vi "Main v1.9.vi"() -> ()   [LabVIEW 2017]
doc: "v0.85:\n- Counts for rejects and total\n\nv0.5:\n\n- Added Reject to Manual Mode\n- Send reject pallet cluster during manual mode\n- Run continuous manual happens only when no error has occured"
uses:
  Controls/Main Tabs v0.1.ctl
  Controls/Auto.ctl
  RT/Controls/Auto Delays.ctl
  RT/Controls/Auto Times.ctl
  support/Controls/General Para.ctl
  Controls/UI Data.ctl
  Controls/AVL Auto Time.ctl
  support/Controls/Auto Stats.ctl
  Controls/Logging FGV.ctl
  support/Message Queue/Enqueue Message (Single).vi
  GV/Maintenance GV.vi
  <vilib>/Utility/error.llb/Error Cluster From Error Code.vi
  <vilib>/ErrorRing/Error Ring.xnode
  support/Message Queue/Message Queue.lvlib
  support/User Event - Stop/User Event - Stop.lvlib
panel:
  out "Rejects 2":u32 caption="Rejects"
  in  "Reset MCount":bool
  out "Output Count":u32 caption="Output\nCount"
  out "OEE":dbl format="%#.1f"
  out "QUA":dbl=100.0 min=0.0 max=100.0 step=0.1
  in  "Ideal Time":dbl=2.0 min=0.0 max=100.0 step=0.1
  in  "AVL":dbl=100.0 min=0.0 max=100.0 step=0.1
  out "PRF":dbl=100.0 min=0.0 max=100.0 step=0.1
  out "path":path
  in  "General Para 2":T1={"Max. Cons."=5.0, "Offset 1"=0.0, "Offset 2"=0.0, "Offset 3"=0.0, "Offset 4"=-0.6, "OutputPause"=500.0, "RejectPause"=500.0} caption="General Para" {"Offset 4" format="%.2f"; "Offset 3" format="%.2f"; "Offset 2" format="%.2f"; "Offset 1" format="%.2f"}
  in  "Auto Para 2":T2={"Agitator Delays"=[250, 600], "TF Delays"=[400, 800, 2, 8000], "Insertion Delays"=[100, 400], "Cutting Delays"=[200, 300, 50], "PF Delays"=[300, 8000], "Measur. Delays"=[200.0, 188.9, 1.0], "Reject Delays"=[500], "BF Delays"=[1000, 1000]}
  out "Shutdown?":bool
  in  "Reject Pallets":T3
  out "Date-Time":string caption="Dip-Tube Assembly Automation (HMI) v1.6"
  out "Main Tab":T4
  in  "All IOs":bool
  in  "Autocycle":T5
  in  "Manual":bool
  in  "Parameters":bool
  in  "Maintenance":bool
  in  "General Para":T1={"Max. Cons."=5.0, "Offset 1"=0.0, "Offset 2"=0.0, "Offset 3"=0.0, "Offset 4"=0.0, "OutputPause"=0.0, "RejectPause"=0.0} {"Offset 4" format="%.2f"; "Offset 3" format="%.2f"; "Offset 2" format="%.2f"; "Offset 1" format="%.2f"}
  in  "BF Para":cluster{"Delay 1":u32, "Delay 2":u32}={"Delay 1"=1000, "Delay 2"=1000}
  in  "Reject Para":cluster{"Delay":u32}={"Delay"=400}
  in  "PF Para":cluster{"Delay 1":u32, "Delay 2":u32}={"Delay 1"=1000, "Delay 2"=1000}
  in  "Tube Feeder Para":T6={"Delay"=400, "Delay 2"=250, "Max Attempts"=250, "Timeout"=8000} caption="TF Para"
  in  "Agitator Para":cluster{"Delay 1":u32, "Delay 2":u32}={"Delay 1"=400, "Delay 2"=250}
  in  "Insertion Para":cluster{"Delay 1":u32, "Delay 2":u32}={"Delay 1"=1000, "Delay 2"=1000}
  in  "Save Para":bool
  in  "Home Para":bool
  in  "Cutting Para":T7={"Delay"=400, "Delay 2"=250, "Delay 3"=250}
  in  "Meas. Para":T8={"Delay"=500.0, "Mean Length"=188.9, "Tolerance"=1.0}
  in  "Enable BF?":bool
  in  "Enable Agitate?":bool
  in  "Enable Reject?":bool
  in  "Toggle Motor":bool
  in  "Continuous?":bool
  in  "Enable Measure?":bool
  in  "Enable Index?":bool
  in  "Enable PF?":bool
  in  "Manual Para":T2={"Agitator Delays"=[400, 250], "TF Delays"=[700, 800, 2], "Insertion Delays"=[100, 500], "Cutting Delays"=[300, 300, 100], "PF Delays"=[250, 30000], "Measur. Delays"=[500.0, 188.9, 1.0], "Reject Delays"=[500], "BF Delays"=[1000, 1000]}
  in  "Enable Cutting?":bool
  in  "Enable Insertion?":bool
  in  "Run Manual":bool
  in  "Enable TF?":bool
  in  "Home Manual":bool
  out "Status 2":T10
  out "Measurements":T11 {"Height 1" format="%#.2f"; "Height 2" format="%#.2f"; "Height 3" format="%#.2f"; "Height 4" format="%#.2f"}
  in  "ResetRejectCount":bool
  in  "ResetGoodCount":bool
  out "RejectPause":u32 caption="Reject Parts"
  out "GoodPause":u32 caption="Good Parts"
  in  "End Cycle":bool
  out "Statuses":string[][](table)
  in  "All IO":bool
  in  "Stats":bool
  in  "Home AC":bool
  out "Status":string
  out "Good":u32 format="%06.0f"
  out "Cycle Time":dbl format="%0.2f"
  out "Rejects":u32 format="%05.0f"
  in  "View Log":bool
  out "Total Count 2":u32 caption="Total Count"
  out "Avg. Time":dbl caption="Avg. Cycle Time (s)" format="%#.3f"
  out "Output Chart":cluster{"Good Parts":u32, "Reject Parts":u32}(graph)
  out "Reject Count":u32
  out "Good Count":u32
  out "Total Time":dbl caption="Effective Cycle Time (s)" format="%#.3f"
  out "Time Chart":T12(graph)
  out "OEE Chart":T13(graph)
  out "Timestamp":string caption="Date & Timestamp"
  out "Latest Measure.":T14 caption="Latest Measurements" {"Length 1 (mm)" format="%#.2f"}
  out "Auto Times":T9
  in  "Back Stats":bool
  out "OEE 2":T13 caption="Latest Measurements" {"AVL" format="%#.1f"; "PRF" format="%#.1f"; "QUA" format="%#.1f"; "OEE" format="%#.1f"}
  out "Measurement Chart":T15(graph)
  in  "Home IOs":bool
  in  "Back IO":bool
  out "IAS 4":dbl format="%#.3f"
  out "IAS 3":dbl format="%#.3f"
  out "IAS 2":dbl format="%#.3f"
  out "IAS 1":dbl format="%#.3f"
  out "DI 1":T16
  out "DI 2":T17
  out "DO 1":T18
  in  "Exit":bool
  in  "Shutdown":bool
  # "HARMONY VISION DIP-TUBE ASSEMBLY AUTOMATION"
  # "Info"
  # "Delays: Time to wait (in milliseconds) after each action pertaining to each spcific station. Generally this timer starts after the required sensor that is expected either goes OFF or goes ON depending on the action. Some stations have multiple delays which are denoted by numbers relative to the sequence of action before the delay.\n\nTimeout: Maximum time allowed (in milliseconds) for a station to complete its actions.\n\nMax Attempts: Maximum number of attempts at retrying gate open/close.\n\nMean Length: Mean length of parts in the current model (in mm)\n\nTolerance: Acceptable deviation from mean length (in mm)\n\nMax Cons.: Maximum number of consecutive tubes missing on a particular pallet (as detected on measurement station) that will trigger an error and cycle stop.\n\nOffset: Offset factor (in mm) added to the measurement result of each probe.\n\nOutputPause & RejectPause: Countdown of number of parts before triggering an Auto-Pause."
  # "Auto-Pause after"
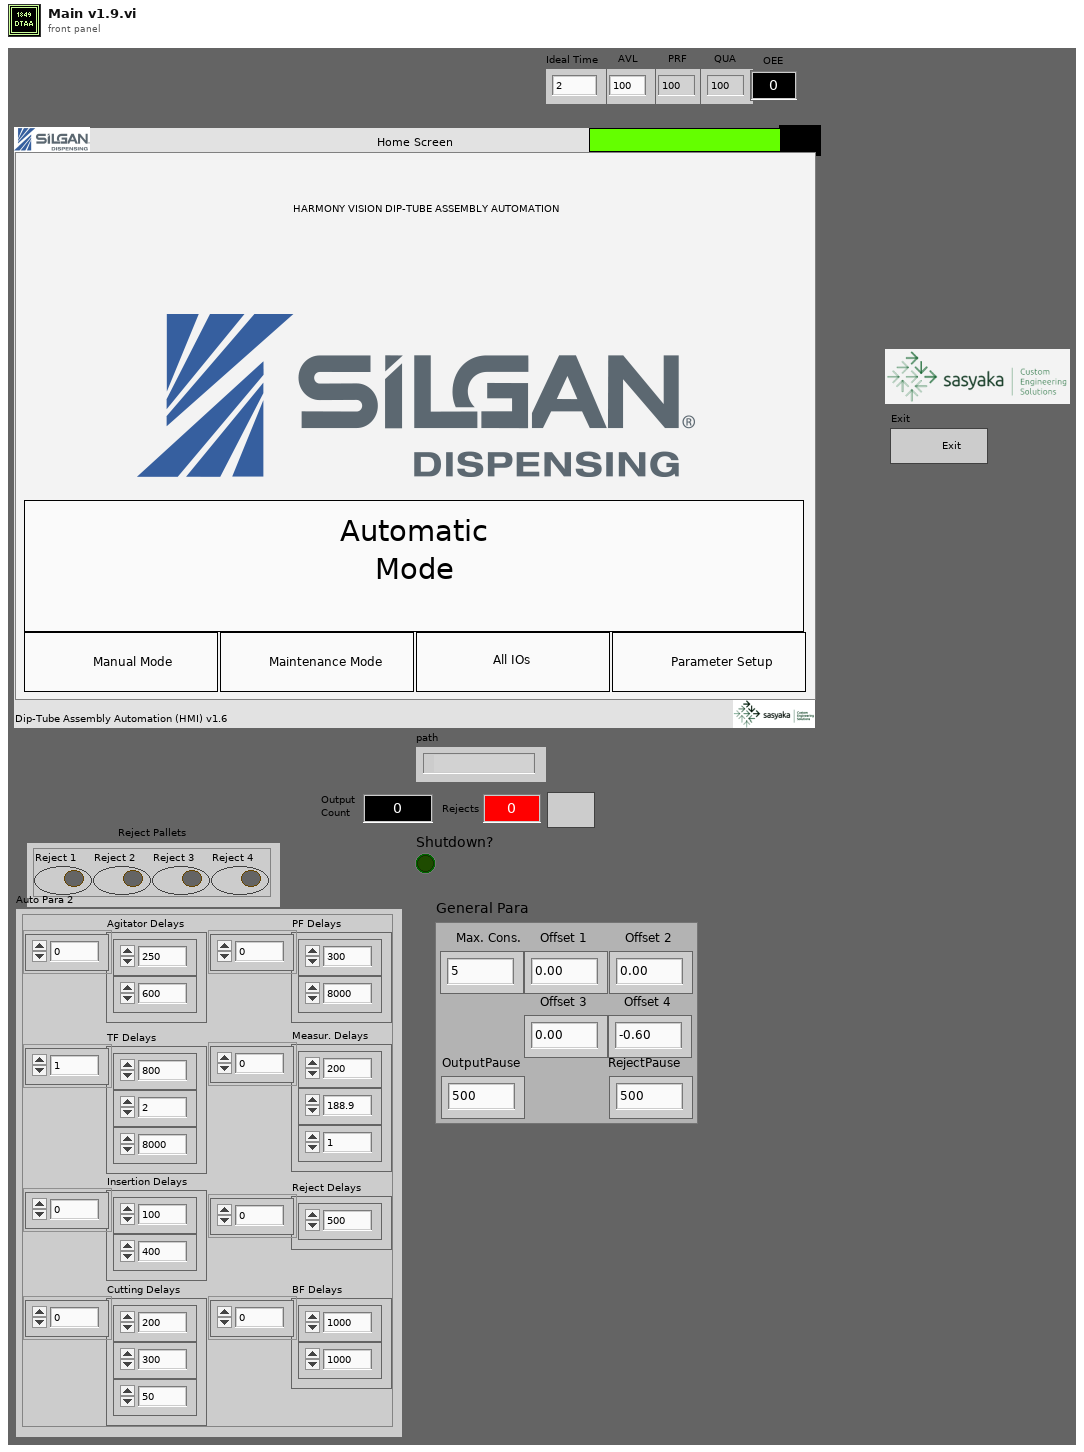
[diagram p1: front panel]
types:
  T1 = typedef "General Para.ctl" = cluster{"Max. Cons.":dbl, "Offset 1":dbl, "Offset 2":dbl, "Offset 3":dbl, "Offset 4":dbl, "OutputPause":dbl, "RejectPause":dbl}
  T2 = typedef "Auto Delays.ctl" = cluster{"Agitator Delays":u32[], "TF Delays":u32[], "Insertion Delays":u32[], "Cutting Delays":u32[], "PF Delays":u32[], "Measur. Delays":dbl[], "Reject Delays":u32[], "BF Delays":u32[]}
  T3 = cluster{"Reject 1":bool, "Reject 2":bool, "Reject 3":bool, "Reject 4":bool}
  T4 = typedef "Main Tabs v0.1.ctl" = enum32{"Home Screen", "Parameter Setup", "Manual Mode", "Autocycle", "Autocycle Statistics", "Autocycle IOs"}
  T5 = typedef "Auto.ctl" = bool
  T6 = cluster{"Delay":u32, "Delay 2":u32, "Max Attempts":u32, "Timeout":u32}
  T7 = cluster{"Delay":u32, "Delay 2":u32, "Delay 3":u32}
  T8 = cluster{"Delay":dbl, "Mean Length":dbl, "Tolerance":dbl}
  T9 = typedef "Auto Times.ctl" = cluster{"Index Time":u32, "TF Time":u32, "Insertion Time":u32, "Cutting Time":u32, "PF Time":u32, "Meas. Time":u32, "Reject Time":u32}
  T10 = cluster{"Auto Times":T9, "error out":errorcluster}
  T11 = cluster{"Height 1":dbl, "Height 2":dbl, "Height 3":dbl, "Height 4":dbl}
  T12 = cluster{"Index":dbl, "TF":dbl, "Insert":dbl, "Cutting":dbl, "PF":dbl, "Measure.":dbl, "Reject":dbl, "Avg. Cycle Time":dbl}
  T13 = cluster{"AVL":dbl, "PRF":dbl, "QUA":dbl, "OEE":dbl}
  T14 = cluster{"Length 1 (mm)":dbl, "Pallet 2 (mm)":dbl, "Pallet 3 (mm)":dbl, "Pallet 4 (mm)":dbl}
  T15 = cluster{"1":dbl, "2":dbl, "3":dbl, "4":dbl, "4":dbl, "4":dbl}
  T16 = cluster{"Machine_ON":bool, "E_stop ":bool, "SW_Pressure":bool, "SW_Start ":bool, "SW_Reset":bool, "SW_Stop":bool, "SW_Door":bool, "RS_Index_Rotary_CW":bool, "RS_Index_Rotary_CCW":bool, "RS_Index_Stopper _Rear":bool, "RS_Index_Output_Separator_Rear":bool, "PES_Index_Pallet_Sensor":bool, "PES_Index_Output_Part Sensor":bool, "ICS_BF_Low_Level_1":bool, "ICS_BF_Low_Level_2":bool, "ICS_BF_Pump_CNVR_Full_1":bool, "ICS_BF_Pump_CNVR_Full_2":bool, "ICS_BF_Pump_CNVR_Full_3":bool, "ICS_BF_Pump_CNVR_Full_4":bool, "PES_PC_Pump Presence_1":bool, "PES_PC_Pump Presence_2":bool, "PES_PC_Pump Presence_3":bool, "PES_PC_Pump Presence_4":bool, "RS_PC_Gating_Front":bool, "PES_Pump_Interference":bool, "PES_TF_Low_Level":bool, "PES_Tube Presence_1":bool, "PES_Tube Presence_2":bool, "PES_Tube Presence_3":bool, "PES_Tube Presence_4":bool, "DI1.30":bool, "DI1.31":bool}
  T17 = cluster{"RS_Agitatator_1_Rear ":bool, "RS_Agitatator_2_Rear ":bool, "RS_TF_Gating CYL_Rear":bool, "RS_Insertion_1_Rear":bool, "RS_Insertion_1_Front":bool, "RS_Insertion _2_Rear":bool, "RS_Insertion _2_Front":bool, "RS_Insertion _3_Rear":bool, "RS_Insertion _3_Front":bool, "RS_Insertion _4_Rear":bool, "RS_Insertion _4_Front":bool, "RS_Insertion_Clamp_Rear":bool, "RS_Cutting_Rear":bool, "RS_Cutting_Clamp _Rear":bool, "RS_Measurement_1_Rear":bool, "RS_Measurement_2_Rear":bool, "RS_Measurement_3_Rear":bool, "RS_Measurement_4_Rear":bool, "DI2.18":bool, "RS_Rejection_1_Rear":bool, "RS_Rejection_2_Rear":bool, "RS_Rejection_3_Rear":bool, "RS_Rejection_4_Rear":bool, "DI2.23":bool, "DI2.24":bool, "DI2.25":bool, "DI2.26":bool, "DI2.27":bool, "DI2.28":bool, "DI2.29":bool, "DI2.30":bool, "DI2.31":bool}
  T18 = cluster{"TL_Red":bool, "TL_Orange":bool, "TL_Green":bool, "TL_Buzzer":bool, "SOL_Index_Rotary_CW":bool, "SOL_Index_Rotary_CCW":bool, "SOL_Index_Stopper_Rear":bool, "SOL_OutputSeparator_Rear":bool, "Bowl  Feeder_ ON 1":bool, "Pump_CNVR_Motor _ON":bool, "SOL_PC_Gating_CYL_Rear":bool, "SOL_Tube_Feed_Agitatator":bool, "SOL_Tube_Feed_Gating_CYL":bool, "SOL_Insertion _CYL":bool, "SOL_Insertion_Clamp_CYL":bool, "SOL_Cutting_CYL":bool, "SOL_Cutting_Clamp_CYL":bool, "SOL_Insertion_Air_Nozzle":bool, "SOL_Measurement_CYL":bool, "DO1.19":bool, "SOL_Rejection CYL_1":bool, "SOL_Rejection CYL_2":bool, "SOL_Rejection CYL_3":bool, "SOL_Rejection CYL_4":bool, "Bowl  Feeder_ ON 2":bool, "SOL_BF_BlowerON":bool, "SOL_BF1_Track1":bool, "SOL_BF1_Track2":bool, "SOL_BF2_Track1":bool, "SOL_BF2_Track2":bool, "DO1.30":bool, "DO1.31":bool}
  T19 = typedef "UI Data.ctl" = cluster{"Main Tab":refnum<vi>}
  T20 = typedef "Message Queue.lvlib/All Message Queues.ctl" = cluster{"UI":refnum<queue>}
  T21 = enum8{"Enabled", "Disabled", "Disabled and Grayed Out"}
  T22 = typedef "AVL Auto Time.ctl" = enum16{"Start Session", "Exited Auto", "Resumed Auto", "Read Time"}
  T23 = cluster{"Array":string[][], "Machine Status":string}
  T24 = typedef "Logging FGV.ctl" = enum16{"Start Shift", "Log Index", "Read Shift", "Close Shift"}
  T25 = typedef "Auto Stats.ctl" = cluster{"Time-Stamp":timestamp, "Auto Times":T9, "Measurements":cluster{"1":dbl, "2":dbl, "3":dbl, "4":dbl}, "Outputs":cluster{"Good Parts":u32, "Reject Parts":u32}, "Cycle Time":dbl, "Remarks":string}
  T26 = cluster{"Auto Times":T9, "Results":cluster{"Measurements":cluster{"1":dbl, "2":dbl, "3":dbl, "4":dbl}, "Reject Pallets":cluster{"Reject 1":bool, "Reject 2":bool, "Reject 3":bool, "Reject 4":bool}}, "OutputCount":u32, "error out":errorcluster}
  T27 = enum8{"Information", "Error", "Successful", "Tips"}
  T28 = cluster{"Agitator Delays[0]":u32, "Agitator Delays[1]":u32}
  T29 = cluster{"TF Delays[0]":u32, "TF Delays[1]":u32, "TF Delays[2]":u32, "TF Delays[3]":u32}
  T30 = cluster{"Insertion Delays[0]":u32, "Insertion Delays[1]":u32}
  T31 = cluster{"Cutting Delays[0]":u32, "Cutting Delays[1]":u32, "Cutting Delays[2]":u32}
  T32 = cluster{"Measur. Delays[0]":dbl, "Measur. Delays[1]":dbl, "Measur. Delays[2]":dbl}
  T33 = typedef "All Inputs.ctl" = cluster{"DI 1":cluster{"Machine_ON":bool, "E_stop ":bool, "SW_Pressure":bool, "SW_Start ":bool, "SW_Reset":bool, "SW_Stop":bool, "SW_Door":bool, "RS_Index_Rotary_CW":bool, "RS_Index_Rotary_CCW":bool, "RS_Index_Stopper _Rear":bool, "RS_Cutting_DNClamp _Rear":bool, "PES_Index_Pallet_Sensor":bool, "PES_Index_Output_Part Sensor":bool, "ICS_BF_Low_Level_1":bool, "ICS_BF_Low_Level_2":bool, "ICS_BF_Pump_CNVR_Full_1":bool, "ICS_BF_Pump_CNVR_Full_2":bool, "ICS_BF_Pump_CNVR_Full_3":bool, "ICS_BF_Pump_CNVR_Full_4":bool, "PES_PC_Pump Presence_1":bool, "PES_PC_Pump Presence_2":bool, "PES_PC_Pump Presence_3":bool, "PES_PC_Pump Presence_4":bool, "RS_PC_Gating_Front":bool, "PES_Pump_Interference":bool, "PES_TF_Low_Level":bool, "PES_Tube Presence_1":bool, "PES_Tube Presence_2":bool, "PES_Tube Presence_3":bool, "PES_Tube Presence_4":bool, "DI1.30":bool, "DI1.31":bool}, "DI 2":cluster{"RS_Agitatator_1_Rear ":bool, "RS_Agitatator_2_Rear ":bool, "RS_TF_Gating CYL_Rear":bool, "RS_Insertion_1_Rear":bool, "RS_Insertion_1_Front":bool, "RS_Insertion _2_Rear":bool, "RS_Insertion _2_Front":bool, "RS_Insertion _3_Rear":bool, "RS_Insertion _3_Front":bool, "RS_Insertion _4_Rear":bool, "RS_Insertion _4_Front":bool, "RS_Insertion_Clamp_Rear":bool, "RS_Cutting_Rear":bool, "RS_Cutting_UPClamp _Rear":bool, "RS_Measurement_1_Rear":bool, "RS_Measurement_2_Rear":bool, "RS_Measurement_3_Rear":bool, "RS_Measurement_4_Rear":bool, "RS_Measure_Clamp_Rear":bool, "RS_Rejection_1_Rear":bool, "RS_Rejection_2_Rear":bool, "RS_Rejection_3_Rear":bool, "RS_Rejection_4_Rear":bool, "DI2.23":bool, "DI2.24":bool, "DI2.25":bool, "DI2.26":bool, "DI2.27":bool, "DI2.28":bool, "DI2.29":bool, "DI2.30":bool, "DI2.31":bool}, "IAS 1":dbl, "IAS 2":dbl, "IAS 3":dbl, "IAS 4":dbl, "DO 1":cluster{"TL_Red":bool, "TL_Orange":bool, "TL_Green":bool, "TL_Buzzer":bool, "SOL_Index_Rotary_CW":bool, "SOL_Index_CNVR_Rotary_CCW":bool, "SOL_Index_CNVR_Stopper_Rear":bool, "SOL_Index_CNVR_Output _Separator _Rear":bool, "Bowl  Feeder_ ON 1":bool, "Pump_CNVR_Motor _ON":bool, "SOL_PC_Gating_CYL_Rear":bool, "SOL_Tube_Feed_Agitatator":bool, "SOL_Tube_Feed_Gating_CYL":bool, "SOL_Insertion _CYL":bool, "SOL_Insertion_Clamp_CYL":bool, "SOL_Cutting_CYL":bool, "SOL_Cutting_Clamp_CYL":bool, "SOL_Insertion_Air_Nozzle":bool, "SOL_Measurement_CYL":bool, "DO1.19":bool, "SOL_Rejection CYL_1":bool, "SOL_Rejection CYL_2":bool, "SOL_Rejection CYL_3":bool, "SOL_Rejection CYL_4":bool, "Bowl  Feeder_ ON 2":bool, "SOL_BF_BlowerON":bool, "SOL_BF1_Track1":bool, "SOL_BF1_Track2":bool, "SOL_BF2_Track1":bool, "SOL_BF2_Track2":bool, "DO1.30":bool, "DO1.31":bool}}
  T34 = cluster{"Machine_ON":bool, "E_stop ":bool, "SW_Pressure":bool, "SW_Start ":bool, "SW_Reset":bool, "SW_Stop":bool, "SW_Door":bool, "RS_Index_Rotary_CW":bool, "RS_Index_Rotary_CCW":bool, "RS_Index_Stopper _Rear":bool, "RS_Cutting_DNClamp _Rear":bool, "PES_Index_Pallet_Sensor":bool, "PES_Index_Output_Part Sensor":bool, "ICS_BF_Low_Level_1":bool, "ICS_BF_Low_Level_2":bool, "ICS_BF_Pump_CNVR_Full_1":bool, "ICS_BF_Pump_CNVR_Full_2":bool, "ICS_BF_Pump_CNVR_Full_3":bool, "ICS_BF_Pump_CNVR_Full_4":bool, "PES_PC_Pump Presence_1":bool, "PES_PC_Pump Presence_2":bool, "PES_PC_Pump Presence_3":bool, "PES_PC_Pump Presence_4":bool, "RS_PC_Gating_Front":bool, "PES_Pump_Interference":bool, "PES_TF_Low_Level":bool, "PES_Tube Presence_1":bool, "PES_Tube Presence_2":bool, "PES_Tube Presence_3":bool, "PES_Tube Presence_4":bool, "DI1.30":bool, "DI1.31":bool}
  T35 = cluster{"RS_Agitatator_1_Rear ":bool, "RS_Agitatator_2_Rear ":bool, "RS_TF_Gating CYL_Rear":bool, "RS_Insertion_1_Rear":bool, "RS_Insertion_1_Front":bool, "RS_Insertion _2_Rear":bool, "RS_Insertion _2_Front":bool, "RS_Insertion _3_Rear":bool, "RS_Insertion _3_Front":bool, "RS_Insertion _4_Rear":bool, "RS_Insertion _4_Front":bool, "RS_Insertion_Clamp_Rear":bool, "RS_Cutting_Rear":bool, "RS_Cutting_UPClamp _Rear":bool, "RS_Measurement_1_Rear":bool, "RS_Measurement_2_Rear":bool, "RS_Measurement_3_Rear":bool, "RS_Measurement_4_Rear":bool, "RS_Measure_Clamp_Rear":bool, "RS_Rejection_1_Rear":bool, "RS_Rejection_2_Rear":bool, "RS_Rejection_3_Rear":bool, "RS_Rejection_4_Rear":bool, "DI2.23":bool, "DI2.24":bool, "DI2.25":bool, "DI2.26":bool, "DI2.27":bool, "DI2.28":bool, "DI2.29":bool, "DI2.30":bool, "DI2.31":bool}
  T36 = cluster{"TL_Red":bool, "TL_Orange":bool, "TL_Green":bool, "TL_Buzzer":bool, "SOL_Index_Rotary_CW":bool, "SOL_Index_CNVR_Rotary_CCW":bool, "SOL_Index_CNVR_Stopper_Rear":bool, "SOL_Index_CNVR_Output _Separator _Rear":bool, "Bowl  Feeder_ ON 1":bool, "Pump_CNVR_Motor _ON":bool, "SOL_PC_Gating_CYL_Rear":bool, "SOL_Tube_Feed_Agitatator":bool, "SOL_Tube_Feed_Gating_CYL":bool, "SOL_Insertion _CYL":bool, "SOL_Insertion_Clamp_CYL":bool, "SOL_Cutting_CYL":bool, "SOL_Cutting_Clamp_CYL":bool, "SOL_Insertion_Air_Nozzle":bool, "SOL_Measurement_CYL":bool, "DO1.19":bool, "SOL_Rejection CYL_1":bool, "SOL_Rejection CYL_2":bool, "SOL_Rejection CYL_3":bool, "SOL_Rejection CYL_4":bool, "Bowl  Feeder_ ON 2":bool, "SOL_BF_BlowerON":bool, "SOL_BF1_Track1":bool, "SOL_BF1_Track2":bool, "SOL_BF2_Track1":bool, "SOL_BF2_Track2":bool, "DO1.30":bool, "DO1.31":bool}
  T37 = cluster{"Index":dbl, "TF":dbl, "Insert":dbl, "Cutting":dbl, "PF":dbl, "Measure.":dbl, "Reject":dbl}
  T38 = cluster{"1":dbl, "2":dbl, "3":dbl, "4":dbl, dbl, dbl}
  T39 = cluster{"Manual Para":T2, "Reject Pallets":cluster{"Reject 1":bool, "Reject 2":bool, "Reject 3":bool, "Reject 4":bool}}
  T40 = cluster{"Measurements":cluster{"1":dbl, "2":dbl, "3":dbl, "4":dbl}, "Reject Pallets":cluster{"Reject 1":bool, "Reject 2":bool, "Reject 3":bool, "Reject 4":bool}}
  T41 = cluster{"Reject Pallets":cluster{"Reject 1":bool, "Reject 2":bool, "Reject 3":bool, "Reject 4":bool}, "Measurements":cluster{"1":dbl, "2":dbl, "3":dbl, "4":dbl}}
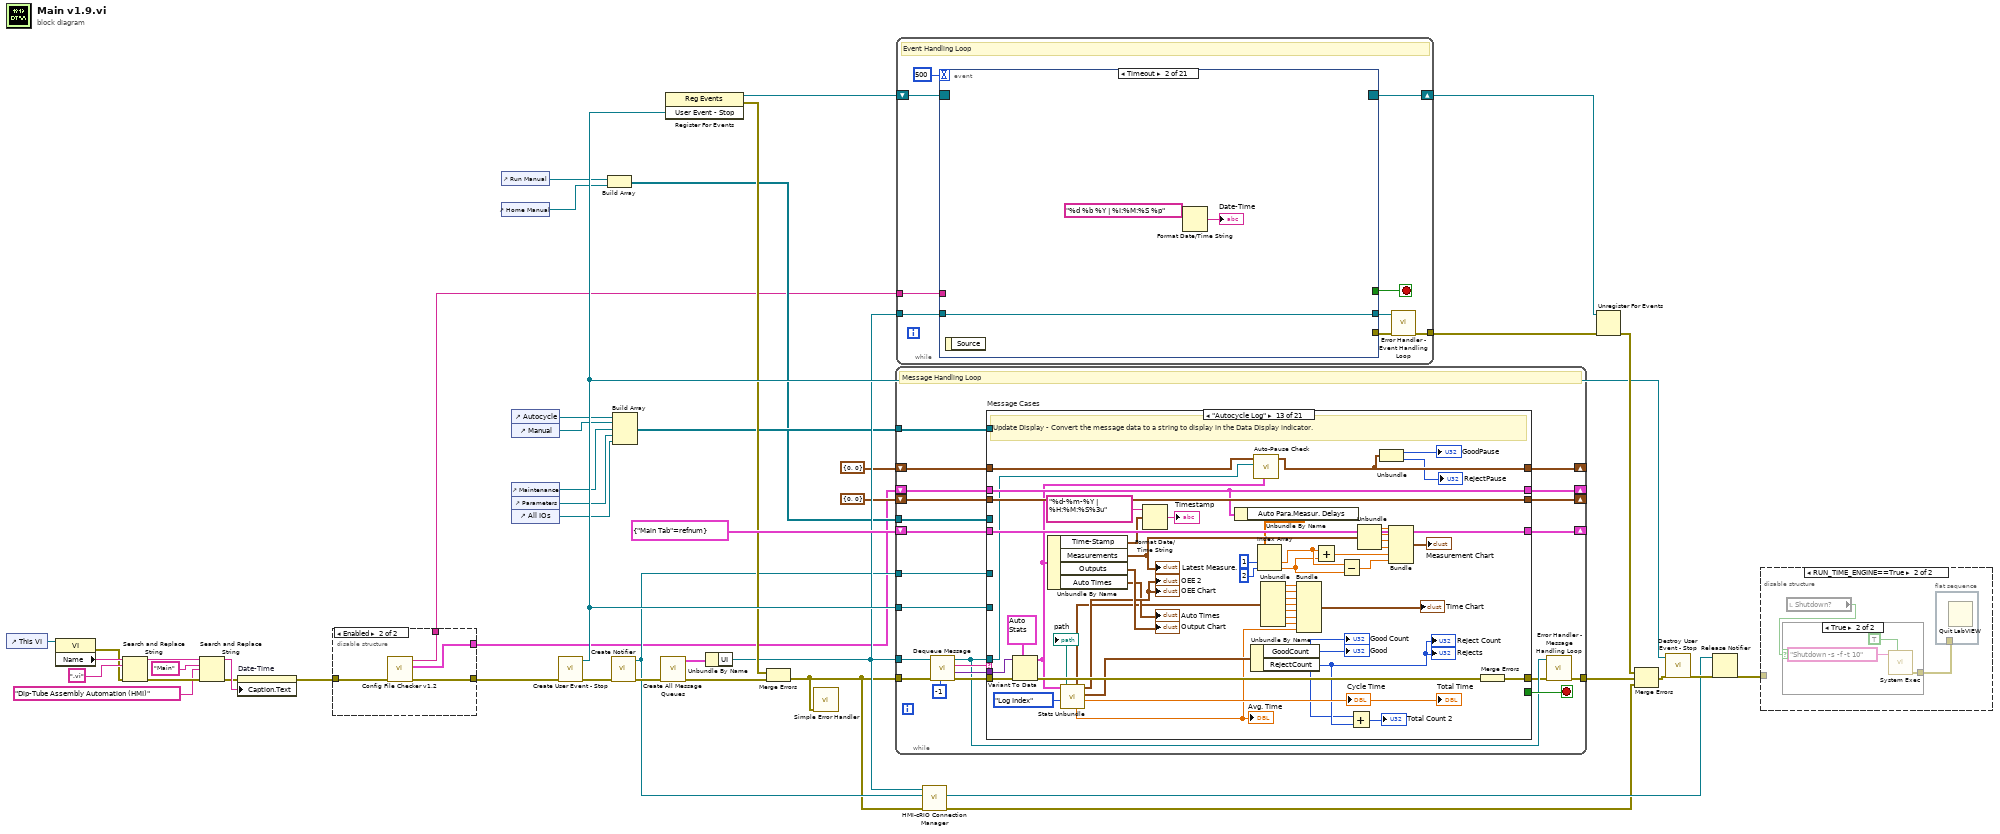
[diagram p0: block diagram]
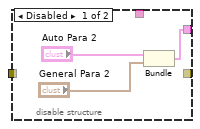
[diagram p2: hidden frame]
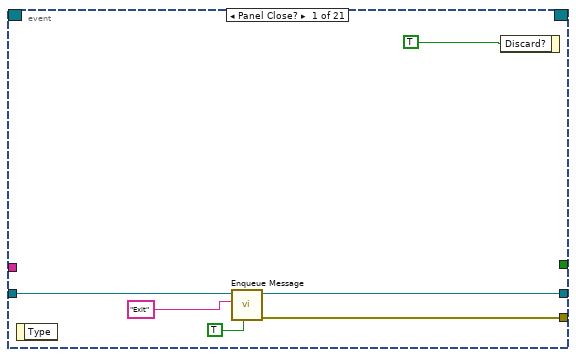
[diagram p3: hidden frame]
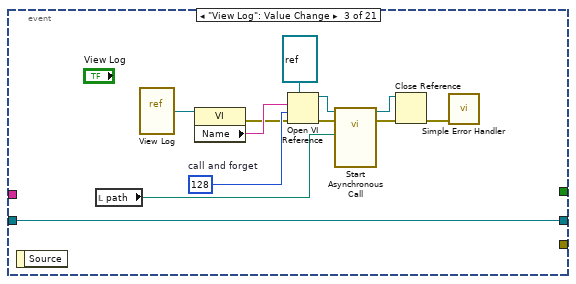
[diagram p4: hidden frame]
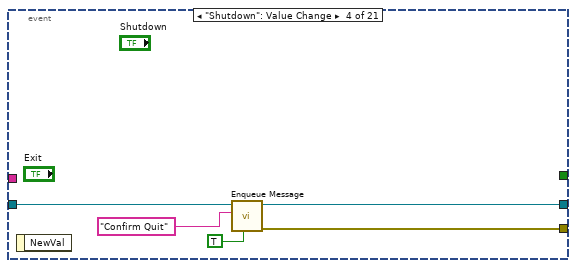
[diagram p5: hidden frame]
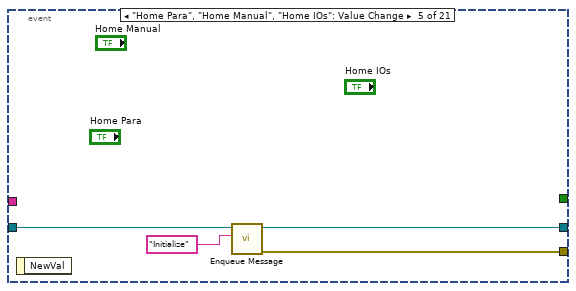
[diagram p6: hidden frame]
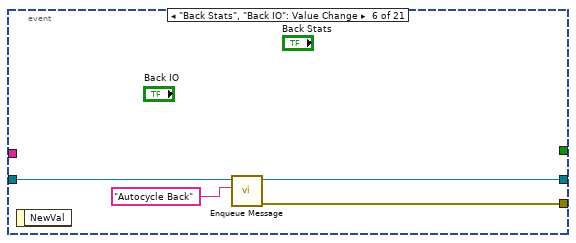
[diagram p7: hidden frame]
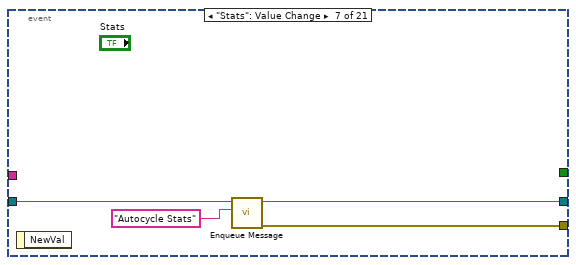
[diagram p8: hidden frame]
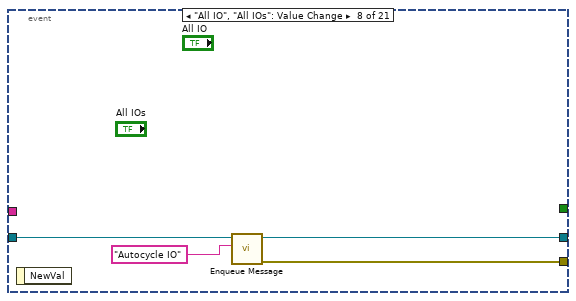
[diagram p9: hidden frame]
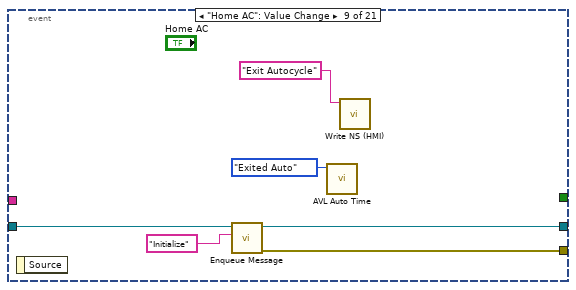
[diagram p10: hidden frame]
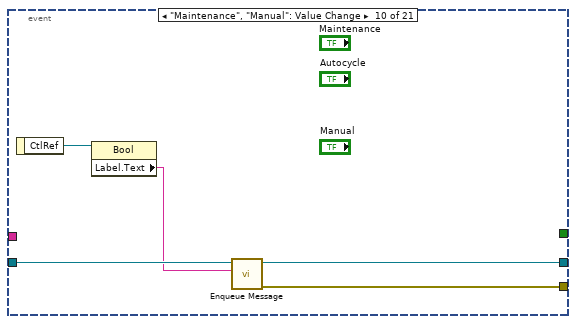
[diagram p11: hidden frame]
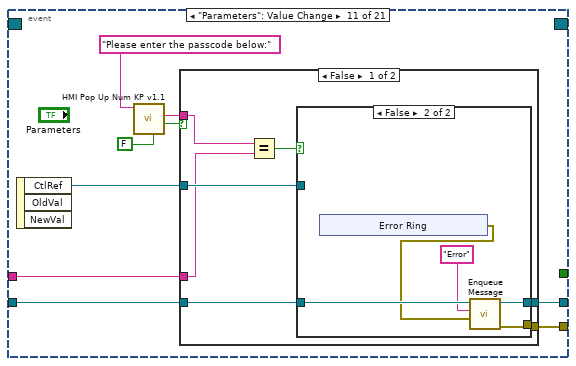
[diagram p12: hidden frame]
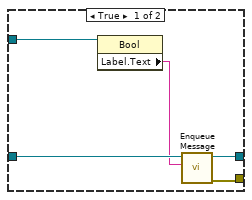
[diagram p13: hidden frame]
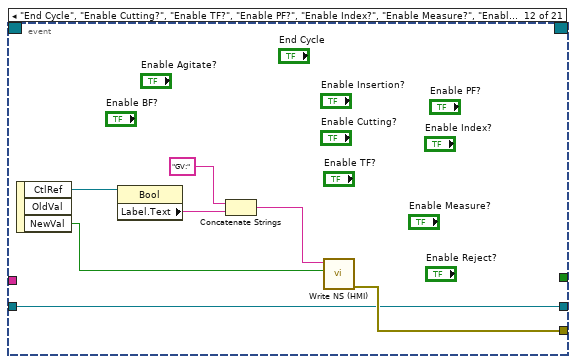
[diagram p15: hidden frame]
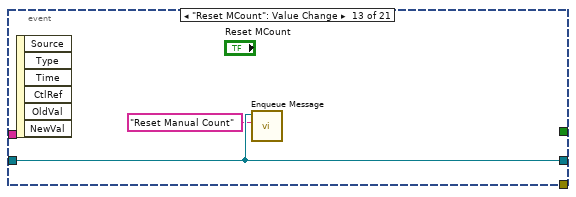
[diagram p16: hidden frame]
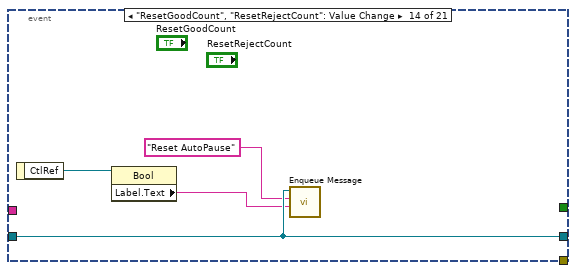
[diagram p17: hidden frame]
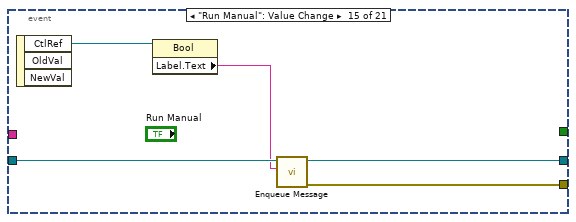
[diagram p18: hidden frame]
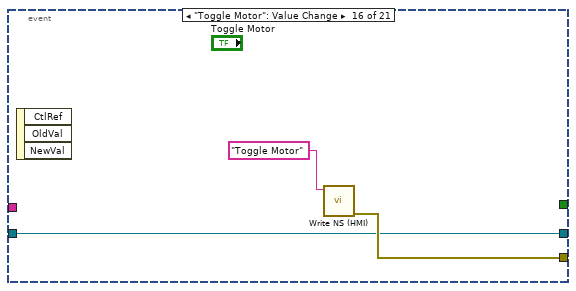
[diagram p19: hidden frame]
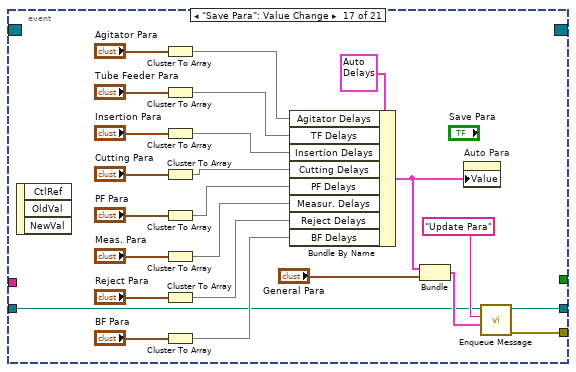
[diagram p20: hidden frame]
diagram:
  n1 = control-ref of="This VI"() -> (w16:refnum<vi>)
  n2 = property class="VI"(reference=w16) -> (error out=w15:errorcluster, "Name"=w22:string)  [unwired: 1 in, 1 out]
  n3 = Search and Replace String(input string=w22, search string=".vi", error in=w15) -> (result string=w20:string, error out=w19:errorcluster)  [unwired: 5 in, 2 out]
  n4 = Search and Replace String(input string=w20, search string="Main", replace string="Dip-Tube Assembly Automation (HMI)" ("replace string (\"\")"), error in=w19) -> (result string=w14:string, error out=w13:errorcluster)  [unwired: 4 in, 2 out]
  n5 = property on="Date-Time" class="Str"(error in=w13, "Caption.Text"=w14) -> (error out=w6:errorcluster)  [unwired: 1 in, 1 out]
  n6 = disable-structure shown="Enabled" {
    disable-tunnel: [w46 w52] -> w4
    disable-tunnel: w6 -> [_ w51]
    disable-tunnel: [_ w50] -> w5
    disable-tunnel: [_ w49] -> w3
    frame Disabled {
      n7 = Bundle("Auto Para 2"="Auto Para 2", "General Para 2"="General Para 2") -> (w46:cluster{"Auto Para 2":T2, "General Para 2":T1})  [unwired: 1 in]
    }
    frame Enabled {
      n8 = call "Config File Checker v1.2.vi"("Error In"=w51) -> ("error out"=w50:errorcluster, "All Para"=w52:cluster{"Auto Para":T2, "General Para 2":T1}, "password"=w49:string)  [unwired: 7 in, 1 out]
    }
  }
  n9 = control-ref of="Run Manual"() -> (w12:refnum<vi>)
  n10 = control-ref of="Home Manual"() -> (w11:refnum<vi>)
  n11 = control-ref of="Autocycle"() -> (w27:refnum<vi>)
  n12 = control-ref of="Manual"() -> (w26:refnum<vi>)
  n13 = control-ref of="Maintenance"() -> (w25:refnum<vi>)
  n14 = control-ref of="Parameters"() -> (w24:refnum<vi>)
  n15 = control-ref of="All IOs"() -> (w7:refnum<vi>)
  n16 = call "Create User Event - Stop.vi"("error in (no error)"=w5) -> ("error out"=w33:errorcluster, "User Event - Stop"=w36:refnum<user-event>)  [unwired: 9 in]
  n17 = Build Array(w12, w11) -> (w10:refnum<vi>[])
  n18 = call "Create Notifier.vi"("error in (no error)"=w33) -> ("error out"=w32:errorcluster, "notifier out"=w8:refnum<notifier>)  [unwired: 9 in]
  n19 = Build Array(w27, w26, w25, w24, w7) -> (w23:refnum<vi>[])
  n20 = call "Create All Message Queues.vi"("error in (no error)"=w32) -> ("error out"=w45:errorcluster, "Message Queues out"=w44:T20)  [unwired: 9 in]
  n21 = register-events(w36) -> (reference out=w37:refnum<event-registration>, error out=w35:errorcluster)  [unwired: 2 in]
  n22 = Unbundle By Name(w44) -> ("UI"=w34:refnum<queue>)
  n23 = Merge Errors(w35, w45) -> (w2:errorcluster)
  n24 = call <vilib>:"Simple Error Handler.vi"("error in (no error)"=w2) -> ()  [unwired: 4 in, 5 out]
  n25 = while {
    tunnel: w34 -> [w67]
    shift-right: [w74] -> _
    shift-left: T19 {"Main Tab"=refnum} ("Data Cluster") -> [w57]
    tunnel: w36 -> [w72]
    tunnel: w2 -> [w71]
    tunnel: [w65] -> w43
    tunnel: w8 -> [w62]
    tunnel: w23 -> [w61]
    tunnel: w10 -> [w60]
    shift-right: [w58] -> _
    shift-left: cluster{"OutputCount":u32, "RejectCount":u32} {"OutputCount"=0, "RejectCount"=0} -> [w59]
    shift-right: [w55] -> _
    shift-left: w4 -> [w56]
    shift-right: [w53] -> _
    shift-left: cluster{"GoodPause":u32, "RejectPause":u32} {"GoodPause"=0, "RejectPause"=0} ("cluster") -> [w54]
    stop <- w73 stop-if-true
    # "Message Handling Loop"
    n26 = call "Dequeue Message.vi"("timeout"=-1, "error in (no error)"=w71, "Message Queue"=w67) -> ("error out"=w70:errorcluster, "Message Data"=w68:variant, "Message"=w69:string, "dup Message Queue"=w66:refnum<queue>)  [unwired: 5 in]
    n27 = case "Message Cases" shown="\"Autocycle Log\"" w69 {
      selector: w69 -> [_ _ _ _ _ _ _ _ _ _ _ _ _ _ _ _ _ _ _ _ w472]
      tunnel: w66 -> [_ _ _ _ _ _ _ _ _ w228 w238 _ w283 _ w364 _ _ _ w441 w468 _]
      tunnel: w70 -> [w84 w89 w105 w135 w152 w170 w181 w214 w221 w230 w246 w276 w326 w338 w372 w384 w394 w431 w445 w461 _]
      tunnel: [w84 w88 w94 w135 w147 w170 w180 w214 w221 w229 w245 w277 w327 w340 w363 w384 w393 w426 w443 w464 w473] -> w64
      tunnel: w57 -> [w83 w90 w107 w139 w154 w169 w177 w218 w225 w235 w243 w278 w328 w341 w373 w383 w396 w430 w444 w467 w474]
      tunnel: [w82 w90 w107 w139 w154 w169 w177 w218 w225 w235 w243 w278 w328 w341 w373 w383 w396 w430 w444 w467 w474] -> w74
      tunnel: [_ _ _ _ _ _ _ _ _ _ _ _ _ _ _ _ _ _ _ TRUE _] -> w73
      tunnel: w68 -> [_ _ w104 _ w151 _ _ _ _ _ _ w275 w325 _ w371 _ w392 w429 _ w458 _]
      tunnel: w72 -> [_ _ _ _ _ _ _ _ _ _ _ _ _ _ _ _ _ _ _ w463 _]
      tunnel: w62 -> [_ _ _ _ _ _ _ _ _ _ _ _ _ _ _ _ _ _ _ w457 _]
      tunnel: w61 -> [_ _ w100 _ _ _ _ _ _ _ _ _ _ _ _ _ _ _ _ _ _]
      tunnel: w60 -> [_ _ _ _ _ _ _ _ _ _ _ _ _ w335 w369 _ _ _ _ _ _]
      tunnel: w59 -> [w79 w87 w96 w136 w153 w158 w182 w215 w222 w232 w247 w273 w323 w331 w362 _ w395 w425 w440 w454 w471]
      tunnel: [w79 w87 w96 w136 w153 w158 w182 w215 w222 w232 w247 w273 w323 w331 w357 cluster{"OutputCount":u32, "RejectCount":u32} {"OutputCount"=0, "RejectCount"=0} w395 w425 w440 w454 w471] -> w58
      tunnel: w56 -> [w76 w86 w93 w116 _ w157 w176 w213 w220 w227 w237 w262 w292 w330 w345 w380 w388 w408 w433 w453 w470]
      tunnel: [w76 w86 w93 w116 w146 w157 w176 w213 w220 w227 w237 w262 w292 w330 w345 w380 w388 w408 w433 w453 w470] -> w55
      tunnel: w54 -> [w75 w85 w91 w115 w140 w155 w173 w212 w219 w226 w236 w261 w284 w329 w344 w379 w389 w407 w432 w452 w469]
      tunnel: [w75 w85 w91 w115 w140 w155 w174 w212 w219 w226 w236 w261 w281 w329 w344 w379 w387 w407 w432 w452 w469] -> w53
      frame "Initialize" {
        # "Initialize - All initialization work should take place in this message, since other loops can potentially enqueue messages that execute immediately after this one."
        n28 = control-ref of="Main Tab"() -> (w81:refnum<vi>)
        n29 = Bundle By Name(cluster=w83, "Main Tab"=w81) -> (w82:T19)
        n30 = property on="Home IOs" class="Bool"("Visible"=TRUE) -> ()  [unwired: 2 in, 2 out]
        n31 = property on="Back IO" class="Bool"("Visible"=FALSE) -> ()  [unwired: 2 in, 2 out]
        "Main Tab" <- Main_Tabs_v0.1."Home Screen" ("Main Tab")
      }
      frame "Maintenance" {
        # "Maintenance"
        n32 = call "Maintenance v0.3.vi"("Error In"=w89) -> ("Error out"=w88:errorcluster)  [unwired: 10 in]
      }
      frame "Connection" {
        n33 = Variant To Data(error in=w105, type=FALSE, Variant=w104) -> (data=w92:bool, error out=w95:errorcluster)
        n34 = Select(t=u32 6618880 ("Text.Text Colors:BG Color"), s=w92, f=u32 16762112 ("Text.Text Colors:BG Color")) -> (s? t:f=w101:u32)
        n35 = property on="Date-Time" class="Str"("Text.BGColor"=w101) -> ()  [unwired: 2 in, 2 out]
        n36 = Select(t=T21."Enabled" ("Disabled"), s=w92, f=T21."Disabled and Grayed Out") -> (s? t:f=w98:T21)
        n37 = for {
          tunnel: w100 -> [w114] mode=indexing
          tunnel: w98 -> [w113]
          n38 = property class="Bool"(reference=w114, "DisabledEnum"=w113) -> ()  [unwired: 1 in, 2 out]
        }
        n39 = case shown="True" w92 {
          tunnel: w95 -> [w108 w111]
          tunnel: [w108 w110] -> w94
          tunnel: w93 -> [_ w109]
          frame False {
          }
          frame True {
            n40 = call "Write NS (HMI).vi"("error in (no error)"=w111, "Message Data"=w109, "Message"="Save Para") -> ("error out"=w110:errorcluster)  [unwired: 8 in]
          }
        }
      }
      frame "Parameters" {
        # "Parameters"
        n41 = Unbundle(w116) -> ("Auto Para"=w118:T2, "General Para 2"=w117:T1)
        n42 = Unbundle By Name(w139) -> ("Main Tab"=w138:refnum<vi>)
        n43 = property on="General Para" class="Clust (strict)"("Value"=w117) -> ()  [unwired: 2 in, 2 out]
        n44 = Unbundle(w118) -> ("Agitator Delays"=w134:u32[], "TF Delays"=w133:u32[], "Insertion Delays"=w132:u32[], "Cutting Delays"=w131:u32[], "PF Delays"=w130:u32[], "Measur. Delays"=w129:dbl[], "Reject Delays"=w128:u32[], "BF Delays"=w127:u32[])
        n45 = property class="TabCtl"(reference=w138, "Value"=Main_Tabs_v0.1."Parameter Setup" ("Main Tab")) -> ()  [unwired: 1 in, 2 out]
        n46 = Array To Cluster(array=w134) -> (cluster=w126:T28)
        n47 = Array To Cluster(array=w133) -> (cluster=w125:T29)
        n48 = Array To Cluster(array=w132) -> (cluster=w124:T30)
        n49 = Array To Cluster(array=w131) -> (cluster=w123:T31)
        n50 = Array To Cluster(array=w130) -> (cluster=w122:cluster{"PF Delays[0]":u32, "PF Delays[1]":u32})
        n51 = Array To Cluster(array=w129) -> (cluster=w121:T32)
        n52 = Array To Cluster(array=w128) -> (cluster=w120:cluster{"Reject Delays[0]":u32})
        n53 = Array To Cluster(array=w127) -> (cluster=w119:cluster{"BF Delays[0]":u32, "BF Delays[1]":u32})
        n54 = property on="Agitator Para" class="Clust (strict)"("Value"=w126) -> ()  [unwired: 2 in, 2 out]
        n55 = property on="Tube Feeder Para" class="Clust (strict)"("Value"=w125) -> ()  [unwired: 2 in, 2 out]
        n56 = property on="Insertion Para" class="Clust (strict)"("Value"=w124) -> ()  [unwired: 2 in, 2 out]
        n57 = property on="Cutting Para" class="Clust (strict)"("Value"=w123) -> ()  [unwired: 2 in, 2 out]
        n58 = property on="PF Para" class="Clust (strict)"("Value"=w122) -> ()  [unwired: 2 in, 2 out]
        n59 = property on="Meas. Para" class="Clust (strict)"("Value"=w121) -> ()  [unwired: 2 in, 2 out]
        n60 = property on="Reject Para" class="Clust (strict)"("Value"=w120) -> ()  [unwired: 2 in, 2 out]
        n61 = property on="BF Para" class="Clust (strict)"("Value"=w119) -> ()  [unwired: 2 in, 2 out]
      }
      frame "Update Para" {
        # "Parameters"
        n62 = Variant To Data(error in=w152, type=cluster{"Auto Para":T2, "General Para":T1} {"Auto Para"={"Agitator Delays"=[], "TF Delays"=[], "Insertion Delays"=[], "Cutting Delays"=[], "PF Delays"=[], "Measur. Delays"=[], "Reject Delays"=[], "BF Delays"=[]}, "General Para"={"Max. Cons."=0.0, "Offset 1"=0.0, "Offset 2"=0.0, "Offset 3"=0.0, "Offset 4"=0.0, "OutputPause"=0.0, "RejectPause"=0.0}} ("cluster"), Variant=w151) -> (data=w146:cluster{"Auto Para":T2, "General Para":T1}, error out=w148:errorcluster)
        n63 = call <vilib>:"Application Directory.vi"() -> ("Application Directory"=w145:path)
        n64 = Build Path(base path=w145, name or relative path="data") -> (appended path=w143:path)
        n65 = Build Path(base path=w143, name or relative path="config.ini") -> (appended path=w142:path)
        n66 = call "Write NS (HMI).vi"("error in (no error)"=w148, "Message Data"=w146, "Message"="Save Para") -> ("error out"=w147:errorcluster)  [unwired: 8 in]
        n67 = call "Write Config v1.1.vi"("All Para"=w146, "file path"=w142) -> ()  [unwired: 8 in, 2 out]
      }
      frame "Manual" {
        # "Parameters"
        n68 = control-ref of="Enable Index?"() -> (w166:refnum<vi>)
        n69 = control-ref of="Enable PF?"() -> (w165:refnum<vi>)
        n70 = control-ref of="Enable Cutting?"() -> (w164:refnum<vi>)
        n71 = control-ref of="Enable Insertion?"() -> (w163:refnum<vi>)
        n72 = control-ref of="Enable TF?"() -> (w162:refnum<vi>)
        n73 = control-ref of="Enable Measure?"() -> (w160:refnum<vi>)
        n74 = Unbundle By Name(w157) -> ("Auto Para"=w156:T2)
        n75 = control-ref of="Enable Reject?"() -> (w159:refnum<vi>)
        n76 = Build Array(w166, w165, w164, w163, w162, w160, w159) -> (w161:refnum<vi>[])
        n77 = property on="Auto Para" class="Clust (strict)"("Value"=w156) -> ()  [unwired: 2 in, 2 out]
        n78 = for {
          tunnel: w161 -> [w172] mode=indexing
          n79 = property class="Bool (strict)"(reference=w172, "Val(Sgnl)"=FALSE ("Value (Signaling)")) -> ()  [unwired: 1 in, 2 out]
        }
        n80 = Unbundle By Name(w169) -> ("Main Tab"=w168:refnum<vi>)
        n81 = property class="TabCtl"(reference=w168, "Value"=Main_Tabs_v0.1."Manual Mode" ("Main Tab")) -> ()  [unwired: 1 in, 2 out]
      }
      frame "Autocycle" {
        # "Parameters"
        n82 = call "Select Model v0.1.vi"() -> ("Cancel out"=w178:bool, "Refresh Indicators?"=w175:bool, "Model out"=w179:string)  [unwired: 9 in]
        n83 = case shown="False" w178 {
          tunnel: w181 -> [w194 w211]
          tunnel: [w201 w211] -> w180
          tunnel: w179 -> [w200 _]
          tunnel: w177 -> [w197 _]
          tunnel: w176 -> [w191 _]
          tunnel: w175 -> [w184 _]
          tunnel: [w188 w210] -> w174
          tunnel: w173 -> [w185 w210]
          frame False {
            n84 = Unbundle By Name(w197) -> ("Main Tab"=w199:refnum<vi>)
            n85 = Unbundle By Name(w191) -> ("General Para 2.OutputPause"=w190:dbl, "General Para 2.RejectPause"=w189:dbl)
            n86 = call "Write NS (HMI).vi"("error in (no error)"=w194, "Message Data"=w191, "Message"="Save Para") -> ("error out"=w193:errorcluster)  [unwired: 8 in]
            n87 = property class="TabCtl"(reference=w199, "Value"=Main_Tabs_v0.1."Autocycle" ("Main Tab")) -> ()  [unwired: 1 in, 2 out]
            n88 = call "Write NS (HMI).vi"("error in (no error)"=w193, "Message Data"=w200, "Message"="Autocycle") -> ("error out"=w201:errorcluster)  [unwired: 8 in]
            n89 = property on="Home IOs" class="Bool"("Visible"=FALSE) -> ()  [unwired: 2 in, 2 out]
            n90 = property on="Back IO" class="Bool"("Visible"=TRUE) -> ()  [unwired: 2 in, 2 out]
            n91 = To Unsigned Long Integer(number=w190) -> (unsigned 32bit integer=w187:u32)
            n92 = To Unsigned Long Integer(number=w189) -> (unsigned 32bit integer=w186:u32)
            n93 = case shown="False" w184 {
              tunnel: [w204 w209] -> w188
              tunnel: w187 -> [_ w207]
              tunnel: w186 -> [_ w206]
              tunnel: w185 -> [w204 w208]
              tunnel: [AVL_Auto_Time."Resumed Auto" ("State") AVL_Auto_Time."Start Session" ("State")] -> w183
              frame False {
              }
              frame True {
                n94 = local write "GoodPause"(w207) -> ()
                n95 = local write "RejectPause"(w206) -> ()
                n96 = Bundle(cluster=w208, "GoodPause"=w207, "RejectPause"=w206) -> (w209:cluster{"GoodPause":u32, "RejectPause":u32})
              }
            }
            n97 = call "AVL Auto Time.vi"("State"=w183) -> ()  [unwired: 10 in, 1 out]
          }
          frame True {
          }
        }
      }
      frame "Autocycle Back" {
        # "Parameters"
        n98 = Unbundle By Name(w218) -> ("Main Tab"=w217:refnum<vi>)
        n99 = property class="TabCtl"(reference=w217, "Value"=Main_Tabs_v0.1."Autocycle" ("Main Tab")) -> ()  [unwired: 1 in, 2 out]
      }
      frame "Autocycle Stats" {
        # "Parameters"
        n100 = Unbundle By Name(w225) -> ("Main Tab"=w224:refnum<vi>)
        n101 = property class="TabCtl"(reference=w224, "Value"=Main_Tabs_v0.1."Autocycle Statistics" ("Main Tab")) -> ()  [unwired: 1 in, 2 out]
      }
      frame "Autocycle IO" {
        # "Parameters"
        n102 = Unbundle By Name(w235) -> ("Main Tab"=w234:refnum<vi>)
        n103 = property class="TabCtl"(reference=w234, "Value"=Main_Tabs_v0.1."Autocycle IOs" ("Main Tab")) -> ()  [unwired: 1 in, 2 out]
        n104 = call-poly "Enqueue Message.vi"("error in (no error)"=w230, "Message"="Update IO", "Message Queue"=w228) -> ("error out"=w229:errorcluster)  [unwired: 7 in, 1 out]
      }
      frame "Update IO" {
        n105 = Unbundle By Name(w243) -> ("Main Tab"=w244:refnum<vi>)
        n106 = Wait (ms)(milliseconds to wait=u32 200) -> ()  [unwired: 1 out]
        n107 = property class="TabCtl"(reference=w244) -> ("Value"=w242:variant)  [unwired: 1 in, 2 out]
        n108 = Variant To Data(type=Main_Tabs_v0.1."Autocycle IOs" ("Main Tab"), Variant=w242) -> (data=w239:T4)  [unwired: 1 in, 1 out]
        n109 = global read "Maintenance GV.vi" "All IO"() -> (w248:T33)
        n110 = case shown="\"Autocycle IOs\"" w239 {
          tunnel: w246 -> [w256 w259]
          tunnel: [w256 w258] -> w245
          tunnel: w238 -> [_ w257]
          frame Default {
          }
          frame "Autocycle IOs" {
            n111 = call-poly "Enqueue Message.vi"("error in (no error)"=w259, "Message"="Update IO", "Message Queue"=w257) -> ("error out"=w258:errorcluster)  [unwired: 7 in, 1 out]
          }
        }
        n112 = Unbundle(w248) -> ("DI 1"=→"DI 1":T34, "DI 2"=→"DI 2":T35, "IAS 1"=→"IAS 1":dbl, "IAS 2"=→"IAS 2":dbl, "IAS 3"=→"IAS 3":dbl, "IAS 4"=→"IAS 4":dbl, "DO 1"=→"DO 1":T36)
      }
      frame "Update UI" {
        # "Update Display - Convert the message data to a string to display in the Data Display indicator."
        n113 = Variant To Data(error in=w276, type=T23 {"Array"=[], "Machine Status"=""} ("Status Cluster"), Variant=w275) -> (data=w271:T23, error out=w274:errorcluster)
        n114 = Unbundle(w271) -> ("Array"=→"Statuses":string[][], "Machine Status"=w269:string)
        "Status" <- w269
        n115 = Search and Replace String(input string=w269, search string="Autocycle is Running") -> (number of replacements=w267:i32)  [unwired: 6 in, 3 out]
        n116 = Greater Than 0?(x=w267) -> (x > 0?=w265:bool)
        n117 = Select(t=T21."Disabled and Grayed Out" ("Disabled"), s=w265, f=T21."Enabled" ("Disabled")) -> (s? t:f=w264:T21)
        n118 = property on="Home AC" class="Bool"("DisabledEnum"=w264) -> ()  [unwired: 2 in, 2 out]
        n119 = Merge Errors(w274) -> (w277:errorcluster)
      }
      frame "Autocycle Log" {
        # "Update Display - Convert the message data to a string to display in the Data Display indicator."
        n120 = Variant To Data(error in=w326, type=T25 {"Time-Stamp"=timestamp(0 s since 1904-01-01), "Auto Times"={"Index Time"=0, "TF Time"=0, "Insertion Time"=0, "Cutting Time"=0, "PF Time"=0, "Meas. Time"=0, "Reject Time"=0}, "Measurements"={"1"=0.0, "2"=0.0, "3"=0.0, "4"=0.0}, "Outputs"={"Good Parts"=0, "Reject Parts"=0}, "Cycle Time"=0.0, "Remarks"=""} ("Auto Stats"), Variant=w325) -> (data=w282:T25, error out=w324:errorcluster)
        n121 = Unbundle By Name(w282) -> ("Time-Stamp"=w320:timestamp, "Measurements"=w312:cluster{"1":dbl, "2":dbl, "3":dbl, "4":dbl}, "Outputs"=→"Output Chart":cluster{"Good Parts":u32, "Reject Parts":u32}, "Auto Times"=→"Auto Times":T9)
        "Latest Measure." <- w312
        n122 = call "Stats Unbundle.vi"("State"=Logging_FGV."Log Index", "Auto Stats"=w282) -> ("Cycle Time"=→"Cycle Time" →"Total Time":dbl, "Counters"=w316:cluster{"GoodCount":u32, "RejectCount":u32}, "OEE Cluster"=→"OEE Chart" →"OEE 2":T13, "Avg. Cycle Time"=w294:dbl, "Total Times"=w302:T37, "path"=→"path":path)  [unwired: 3 in, 1 out]
        "Avg. Time" <- w294
        n123 = Format Date/Time String(time format string (%c)="%d-%m-%Y | %H:%M:%S%3u", seconds (now)=w320) -> (date/time string=→"Timestamp":string)  [unwired: 1 in]
        n124 = Unbundle By Name(w292) -> ("Auto Para.Measur. Delays"=w291:dbl[])
        n125 = Unbundle By Name(w316) -> ("GoodCount"=w304:u32, "RejectCount"=w305:u32)
        "Rejects" <- w305
        "Good" <- w304
        "Good Count" <- w304
        "Reject Count" <- w305
        n126 = call "Auto-Pause Check.vi"("Auto Stats"=w282, "Queue"=w283, "Autopause"=w284) -> ("Autopause out"=w281:cluster{"GoodPause":u32, "RejectPause":u32})  [unwired: 8 in]
        n127 = Index Array(array=w291, index #1=1 ("index"), index #2=2 ("index")) -> (element #1=w286:dbl, element #2=w285:dbl)
        n128 = Unbundle(w302) -> ("Index"=w301:dbl, "TF"=w300:dbl, "Insert"=w299:dbl, "Cutting"=w298:dbl, "PF"=w297:dbl, "Measure."=w296:dbl, "Reject"=w295:dbl)
        n129 = Bundle("Index"=w301, "TF"=w300, "Insert"=w299, "Cutting"=w298, "PF"=w297, "Measure."=w296, "Reject"=w295, "Avg. Cycle Time"=w294) -> (→"Time Chart":T12)  [unwired: 1 in]
        n130 = Add(x=w286, y=w285) -> (x+y=w288:dbl)
        n131 = Subtract(x=w286, y=w285) -> (x-y=w287:dbl)
        n132 = Add(x=w304, y=w305) -> (x+y=→"Total Count 2":u32)
        n133 = Unbundle(w312) -> ("1"=w311:dbl, "2"=w310:dbl, "3"=w309:dbl, "4"=w308:dbl)
        n134 = Unbundle(w281) -> ("GoodPause"=→"GoodPause":u32, "RejectPause"=→"RejectPause":u32)
        n135 = Bundle("1"=w311, "2"=w310, "3"=w309, "4"=w308, w288, w287) -> (→"Measurement Chart":T38)  [unwired: 1 in]
        n136 = Merge Errors(w324) -> (w327:errorcluster)
      }
      frame "Run Manual" {
        # "Update Manual mode"
        n137 = Bundle("Manual Para"="Manual Para", "Reject Pallets"="Reject Pallets") -> (w332:T39)  [unwired: 1 in]
        n138 = for {
          tunnel: w335 -> [w343] mode=indexing
          tunnel: T21."Disabled and Grayed Out" ("Disabled") -> [w342]
          n139 = property class="Bool"(reference=w343, "DisabledEnum"=w342) -> ()  [unwired: 1 in, 2 out]
        }
        n140 = call "Write NS (HMI).vi"("error in (no error)"=w338, "Message Data"=w332, "Message"="Manual Run") -> ("error out"=w337:errorcluster)  [unwired: 8 in]
        n141 = Merge Errors(w337) -> (w340:errorcluster)
      }
      frame "Manual Status" {
        n142 = Variant To Data(error in=w372, type=T26 {"Auto Times"={"Index Time"=0, "TF Time"=0, "Insertion Time"=0, "Cutting Time"=0, "PF Time"=0, "Meas. Time"=0, "Reject Time"=0}, "Results"={"Measurements"={"1"=0.0, "2"=0.0, "3"=0.0, "4"=0.0}, "Reject Pallets"={"Reject 1"=FALSE, "Reject 2"=FALSE, "Reject 3"=FALSE, "Reject 4"=FALSE}}, "OutputCount"=0, "error out"={"status"=FALSE, "code"=0, "source"=""}} ("cluster"), Variant=w371) -> (data=w368:T26, error out=w363:errorcluster)
        n143 = Unbundle(w368) -> ("Auto Times"=w367:T9, "Results"=w359:T40, "OutputCount"=w358:u32, "error out"=w361:errorcluster)
        n144 = for {
          tunnel: w369 -> [w378] mode=indexing
          tunnel: T21."Enabled" ("Disabled") -> [w377]
          n145 = property class="Bool"(reference=w378, "DisabledEnum"=w377) -> ()  [unwired: 1 in, 2 out]
        }
        n146 = Unbundle(w359) -> ("Measurements"=w347:cluster{"1":dbl, "2":dbl, "3":dbl, "4":dbl}, "Reject Pallets"=w348:T3)
        "Measurements" <- w347
        n147 = Bundle("Auto Times"=w367, "error out"=w361) -> (→"Status 2":T10)  [unwired: 1 in]
        n148 = Bundle("Reject Pallets"=w348, "Measurements"=w347) -> (w346:T41)  [unwired: 1 in]
        n149 = call "Counts Update (manual).vi"("output cluster"=w346, "Desired Cycle Time (s)"="Ideal Time", "AVL"="AVL", "OutputCount"=w358, "Counts in"=w362) -> ("OEE"=w352:T13, "Counts out"=w357:cluster{"OutputCount":u32, "RejectCount":u32})  [unwired: 5 in]
        n150 = Unbundle(w352) -> ("PRF"=→"PRF":dbl, "QUA"=→"QUA":dbl, "OEE"=→"OEE":dbl)  [unwired: 1 out]
        n151 = Unbundle(w357) -> ("OutputCount"=→"Output Count":u32, "RejectCount"=→"Rejects 2":u32)
        n152 = case shown="True" "Continuous?" {
          tunnel: w364 -> [_ w376]
          tunnel: w361 -> [_ w375]
          frame False {
          }
          frame True {
            # "Run if continuous is TRUE & No Error"
            n153 = call-poly "Enqueue Message.vi"("error in (no error)"=w375, "Message"="Run Manual", "Message Queue"=w376) -> ()  [unwired: 7 in, 2 out]
          }
        }
      }
      frame "Reset Manual Count" {
        w381 = u32 0 ("Rejects")
        n154 = local write "Rejects 2"(w381) -> ()
        n155 = local write "Output Count"(w381) -> ()
      }
      frame "Reset AutoPause" {
        n156 = Variant To Data(error in=w394, type="" ("Message"), Variant=w392) -> (data=w390:string, error out=w393:errorcluster)
        n157 = case shown="\"ResetRejectCount\", Default" w390 {
          tunnel: w389 -> [w401 w406]
          tunnel: [w400 w405] -> w387
          tunnel: w388 -> [w399 w404]
          frame "ResetGoodCount" {
            n158 = Unbundle By Name(w399) -> ("General Para 2.OutputPause"=w398:dbl)
            n159 = To Unsigned Long Integer(number=w398) -> (unsigned 32bit integer=w397:u32)
            n160 = Bundle By Name(cluster=w401, "GoodPause"=w397) -> (w400:cluster{"GoodPause":u32, "RejectPause":u32})
          }
          frame "ResetRejectCount", Default {
            n161 = Unbundle By Name(w404) -> ("General Para 2.RejectPause"=w403:dbl)
            n162 = To Unsigned Long Integer(number=w403) -> (unsigned 32bit integer=w402:u32)
            n163 = Bundle By Name(cluster=w406, "RejectPause"=w402) -> (w405:cluster{"GoodPause":u32, "RejectPause":u32})
          }
        }
        n164 = Unbundle(w387) -> ("GoodPause"=w386:u32, "RejectPause"=w385:u32)
        n165 = local write "GoodPause"(w386) -> ()
        n166 = local write "RejectPause"(w385) -> ()
      }
      frame "Error" {
        w412 = 128  # call and forget
        # "Run async so that this loop will continue to run"
        # "Error"
        n167 = Variant To Data(error in=w431, type=errorcluster {"status"=FALSE, "code"=0, "source"=""} ("error constant"), Variant=w429) -> (data=w424:errorcluster, error out=w427:errorcluster)
        n168 = Unbundle By Name(w424) -> ("source"=w423:string)
        n169 = vi-ref "NewDialog.vi"() -> (w419:refnum<vi>)
        n170 = property class="VI"(reference=w419) -> (error out=w421:errorcluster, "Name"=w420:string)  [unwired: 1 in, 1 out]
        n171 = Search and Replace String(input string=w423, search string="<err>") -> (result string=w411:string)  [unwired: 6 in, 3 out]
        n172 = Open VI Reference(type specifier VI Refnum (for type only)=refnum<vi> refnum, vi path=w420, options=w412, error in (no error)=w421) -> (vi reference=w414:refnum<vi>, error out=w415:errorcluster)  [unwired: 2 in]
        n173 = call-by-ref "Start Asynchronous Call"(reference=w414, error in=w415, "inIcon"=T27."Error", "inTitle"="ERROR", "inMessage"=w411) -> (reference out=w417:refnum<vi>, error out=w416:errorcluster)  [unwired: 6 in, 3 out]
        n174 = Close Reference(reference=w417, error in (no error)=w416) -> (error out=w418:errorcluster)
        n175 = call <vilib>:"Simple Error Handler.vi"("error in (no error)"=w418) -> ()  [unwired: 4 in, 5 out]
        n176 = Merge Errors(w427) -> (w426:errorcluster)
      }
      frame "Confirm Quit" {
        # "Confirm Quit - Message that can confirm whether or not the user wants to exit the application."
        n177 = call "NewDialog.vi"("inIcon"=T27."Information", "inTitle"="SHUTDOWN?", "inButton2Text"="Shutdown", "inButton1Text"="", "inMessage"="Are you sure you want to shutdown?") -> ("outButton2"=w434:bool)  [unwired: 4 in, 2 out]
        "Shutdown?" <- w434
        n178 = case shown="True" w434 {
          tunnel: w445 -> [w446 w451]
          tunnel: [w446 w450] -> w442
          tunnel: w441 -> [_ w449]
          frame False {
          }
          frame True {
            n179 = call-poly "Enqueue Message.vi"("Priority Message? (F)"=TRUE, "error in (no error)"=w451, "Message"="Exit", "Message Queue"=w449) -> ("error out"=w450:errorcluster)  [unwired: 6 in, 1 out]
          }
        }
        n180 = Merge Errors(w442) -> (w443:errorcluster)
      }
      frame "Exit" {
        # "Stop the VI"
        # "Release the message queue reference"
        # "Exit - Exit the application."
        n181 = Variant To Data(type=errorcluster {"status"=FALSE, "code"=0, "source"=""} ("error constant"), Variant=w458) -> (data=w459:errorcluster)  [unwired: 1 in, 1 out]
        n182 = call <vilib>:"Simple Error Handler.vi"("error in (no error)"=w459) -> ()  [unwired: 4 in, 5 out]
        n183 = Send Notification(notification=TRUE, notifier=w457) -> (error out=w455:errorcluster)  [unwired: 1 in, 1 out]
        n184 = call "Fire User Event - Stop.vi"("User Event - Stop"=w463) -> ("error out"=w462:errorcluster)  [unwired: 10 in]
        n185 = Release Queue(queue=w468, error in (no error)=w461) -> (error out=w465:errorcluster)  [unwired: 1 in, 2 out]
        n186 = Merge Errors(w455, w462, w465) -> (w464:errorcluster)
      }
      frame Default {
        # "'Default' case only runs if there is a message that isn't defined in any of the other cases.  Output a programming error."
        n187 = xnode "Error Ring"("parameter 0"=w472) -> ("error out"=w473:errorcluster)
      }
    }
    n188 = call "Error Handler - Message Handling Loop.vi"("error in (no error)"=w64, "Message Queue"=w66) -> ("dup error in"=w65:errorcluster)  [unwired: 8 in, 1 out]
  }
  n189 = while {
    tunnel: w34 -> [w490]
    shift-right: [w488] -> w40
    shift-left: w37 -> [w489]
    tunnel: [w484] -> w38
    tunnel: w3 -> [w482]
    stop <- w486 stop-if-true
    # "Event Handling Loop"
    n190 = event shown="[1] Timeout" {
      selector: w489 -> [_ _ _ _ _ _ _ _ _ _ _ _ _ _ _ _ _ _ _ _ _]
      dyn-events: [_ _ _ _ _ _ _ _ _ _ _ _ _ _ _ _ _ _ _ _ _] -> w488
      timeout: 500 -> [_ _ _ _ _ _ _ _ _ _ _ _ _ _ _ _ _ _ _ _ _]
      tunnel: [_ _ _ _ _ _ _ _ _ _ _ _ _ _ _ _ _ _ _ _ TRUE ("Discard?")] -> w486
      tunnel: w490 -> [w495 w499 w511 w516 w520 w524 w528 w532 w538 w543 w552 w576 w580 w584 w589 w591 w594 w625 w634 w643 w645]
      tunnel: [w494 _ _ w515 w519 w523 w527 w531 w537 w542 w551 w577 _ _ w587 w592 w597 _ _ _ _] -> w487
      tunnel: [w493 w499 w511 w514 w518 w522 w526 w530 w536 w541 w550 w576 w580 w584 w588 w591 w593 w625 w634 w643 w645] -> w485
      tunnel: w482 -> [_ _ _ _ _ _ _ _ _ _ w544 _ _ _ _ _ _ _ _ _ _]
      event Panel Close? {
        n191 = event-data() -> ()  [unwired: 1 in, 1 out]
        n192 = call-poly "Enqueue Message.vi"("Priority Message? (F)"=TRUE, "Message"="Exit", "Message Queue"=w495) -> ("error out"=w494:errorcluster, "dup Message Queue"=w493:refnum<queue>)  [unwired: 7 in]
        n193 = event-data("Discard?"=TRUE) -> ()  [unwired: 1 in, 1 out]
      }
      event Timeout {
        n194 = event-data() -> ()  [unwired: 1 in, 1 out]
        n195 = Format Date/Time String(time format string (%c)="%d %b %Y | %I:%M:%S %p") -> (date/time string=→"Date-Time":string)  [unwired: 2 in]
      }
      event "View Log": Value Change {
        w510 = 128  # call and forget
        n196 = event-data() -> ()  [unwired: 1 in, 1 out]
        n197 = local read "path"() -> (w500:path)
        n198 = vi-ref "View Log.vi"() -> (w503:refnum<vi>)
        n199 = property class="VI"(reference=w503) -> (error out=w501:errorcluster, "Name"=w502:string)  [unwired: 1 in, 1 out]
        n200 = Open VI Reference(type specifier VI Refnum (for type only)=refnum<vi> refnum, vi path=w502, options=w510, error in (no error)=w501) -> (vi reference=w508:refnum<vi>, error out=w507:errorcluster)  [unwired: 2 in]
        n201 = call-by-ref "Start Asynchronous Call"(reference=w508, error in=w507, "file path"=w500) -> (reference out=w505:refnum<vi>, error out=w506:errorcluster)  [unwired: 10 in, 1 out]
        n202 = Close Reference(reference=w505, error in (no error)=w506) -> (error out=w504:errorcluster)
        n203 = call <vilib>:"Simple Error Handler.vi"("error in (no error)"=w504) -> ()  [unwired: 4 in, 5 out]
      }
      event "Shutdown": Value Change {
        n204 = event-data() -> ()  [unwired: 1 in, 1 out]
        n205 = call-poly "Enqueue Message.vi"("Priority Message? (F)"=TRUE, "Message"="Confirm Quit", "Message Queue"=w516) -> ("error out"=w515:errorcluster, "dup Message Queue"=w514:refnum<queue>)  [unwired: 7 in]
      }
      event "Home Para", "Home Manual", "Home IOs": Value Change {
        n206 = event-data() -> ()  [unwired: 1 in, 1 out]
        n207 = call-poly "Enqueue Message.vi"("Message"="Initialize", "Message Queue"=w520) -> ("error out"=w519:errorcluster, "dup Message Queue"=w518:refnum<queue>)  [unwired: 8 in]
      }
      event "Back Stats", "Back IO": Value Change {
        n208 = event-data() -> ()  [unwired: 1 in, 1 out]
        n209 = call-poly "Enqueue Message.vi"("Message"="Autocycle Back", "Message Queue"=w524) -> ("error out"=w523:errorcluster, "dup Message Queue"=w522:refnum<queue>)  [unwired: 8 in]
      }
      event "Stats": Value Change {
        n210 = event-data() -> ()  [unwired: 1 in, 1 out]
        n211 = call-poly "Enqueue Message.vi"("Message"="Autocycle Stats", "Message Queue"=w528) -> ("error out"=w527:errorcluster, "dup Message Queue"=w526:refnum<queue>)  [unwired: 8 in]
      }
      event "All IO", "All IOs": Value Change {
        n212 = event-data() -> ()  [unwired: 1 in, 1 out]
        n213 = call-poly "Enqueue Message.vi"("Message"="Autocycle IO", "Message Queue"=w532) -> ("error out"=w531:errorcluster, "dup Message Queue"=w530:refnum<queue>)  [unwired: 8 in]
      }
      event "Home AC": Value Change {
        n214 = event-data() -> ()  [unwired: 1 in, 1 out]
        n215 = call-poly "Enqueue Message.vi"("Message"="Initialize", "Message Queue"=w538) -> ("error out"=w537:errorcluster, "dup Message Queue"=w536:refnum<queue>)  [unwired: 8 in]
        n216 = call "AVL Auto Time.vi"("State"=AVL_Auto_Time."Exited Auto") -> ()  [unwired: 10 in, 1 out]
        n217 = call "Write NS (HMI).vi"("Message"="Exit Autocycle") -> ()  [unwired: 10 in, 1 out]
      }
      event "Maintenance", "Manual": Value Change {
        n218 = event-data() -> ("CtlRef"=w540:refnum<vi>)  [unwired: 1 in]
        n219 = property class="Bool"(reference=w540) -> ("Label.Text"=w539:string)  [unwired: 1 in, 2 out]
        n220 = call-poly "Enqueue Message.vi"("Message"=w539, "Message Queue"=w543) -> ("error out"=w542:errorcluster, "dup Message Queue"=w541:refnum<queue>)  [unwired: 8 in]
      }
      event "Parameters": Value Change {
        n221 = event-data() -> ("CtlRef"=w549:refnum<vi>)  [unwired: 1 in, 2 out]
        n222 = call "HMI Pop Up Num KP v1.1.vi"("Password Display (F)"=FALSE, "Message In"="Please enter the passcode below:") -> ("Canceled"=w546:bool, "String Out"=w545:string)  [unwired: 8 in]
        n223 = case shown="False" w546 {
          tunnel: w552 -> [w559 w571]
          tunnel: [w558 _] -> w551
          tunnel: [w557 w571] -> w550
          tunnel: w549 -> [w556 _]
          tunnel: w545 -> [w555 _]
          tunnel: w544 -> [w554 _]
          frame False {
            n224 = Equal?(x=w555, y=w554) -> (x = y?=w553:bool)
            n225 = case shown="False" w553 {
              tunnel: w559 -> [w564 w569]
              tunnel: [w563 w568] -> w558
              tunnel: [w562 w567] -> w557
              tunnel: w556 -> [w561 _]
              frame True {
                n226 = property class="Bool"(reference=w561) -> ("Label.Text"=w560:string)  [unwired: 1 in, 2 out]
                n227 = call-poly "Enqueue Message.vi"("Message"=w560, "Message Queue"=w564) -> ("error out"=w563:errorcluster, "dup Message Queue"=w562:refnum<queue>)  [unwired: 8 in]
              }
              frame False {
                n228 = xnode "Error Ring"() -> ("error out"=w565:errorcluster)
                n229 = call-poly "Enqueue Message.vi"("Message Data"=w565, "Message"="Error" ("Message In"), "Message Queue"=w569) -> ("error out"=w568:errorcluster, "dup Message Queue"=w567:refnum<queue>)  [unwired: 7 in]
              }
            }
          }
          frame True {
          }
        }
      }
      event "End Cycle", "Enable Cutting?", "Enable TF?", "Enable PF?", "Enable Index?", "Enable Measure?", "Enable Reject?", "Enable Agitate?", "Enable BF?", "Enable Insertion?": Value Change {
        n230 = event-data() -> ("CtlRef"=w578:refnum<vi>, "NewVal"=w572:bool)  [unwired: 1 in, 1 out]
        n231 = property class="Bool"(reference=w578) -> ("Label.Text"=w575:string)  [unwired: 1 in, 2 out]
        n232 = Concatenate Strings("GV:" ("string"), w575) -> (w573:string)
        n233 = call "Write NS (HMI).vi"("Message Data"=w572, "Message"=w573) -> ("error out"=w577:errorcluster)  [unwired: 9 in]
      }
      event "Reset MCount": Value Change {
        n234 = event-data() -> ()  [unwired: 1 in, 6 out]
        n235 = call-poly "Enqueue Message.vi"("Message"="Reset Manual Count", "Message Queue"=w580) -> ()  [unwired: 8 in, 2 out]
      }
      event "ResetGoodCount", "ResetRejectCount": Value Change {
        n236 = event-data() -> ("CtlRef"=w582:refnum<vi>)  [unwired: 1 in]
        n237 = property class="Bool"(reference=w582) -> ("Label.Text"=w581:string)  [unwired: 1 in, 2 out]
        n238 = call-poly "Enqueue Message.vi"("Message Data"=w581, "Message"="Reset AutoPause", "Message Queue"=w584) -> ()  [unwired: 7 in, 2 out]
      }
      event "Run Manual": Value Change {
        n239 = event-data() -> ("CtlRef"=w586:refnum<vi>)  [unwired: 1 in, 2 out]
        n240 = property class="Bool"(reference=w586) -> ("Label.Text"=w585:string)  [unwired: 1 in, 2 out]
        n241 = call-poly "Enqueue Message.vi"("Message"=w585, "Message Queue"=w589) -> ("error out"=w587:errorcluster, "dup Message Queue"=w588:refnum<queue>)  [unwired: 8 in]
      }
      event "Toggle Motor": Value Change {
        n242 = event-data() -> ()  [unwired: 1 in, 3 out]
        n243 = call "Write NS (HMI).vi"("Message"="Toggle Motor") -> ("error out"=w592:errorcluster)  [unwired: 10 in]
      }
      event "Save Para": Value Change {
        n244 = event-data() -> ()  [unwired: 1 in, 3 out]
        n245 = Cluster To Array(cluster="Agitator Para") -> (array=w614:u32[])
        n246 = Cluster To Array(cluster="Tube Feeder Para") -> (array=w612:u32[])
        n247 = Cluster To Array(cluster="Insertion Para") -> (array=w610:u32[])
        n248 = Cluster To Array(cluster="Cutting Para") -> (array=w608:u32[])
        n249 = Cluster To Array(cluster="PF Para") -> (array=w606:u32[])
        n250 = Cluster To Array(cluster="Meas. Para") -> (array=w604:dbl[])
        n251 = Cluster To Array(cluster="Reject Para") -> (array=w602:u32[])
        n252 = Cluster To Array(cluster="BF Para") -> (array=w600:u32[])
        n253 = Bundle By Name(cluster=T2 {"Agitator Delays"=[1000], "TF Delays"=[1000], "Insertion Delays"=[1000], "Cutting Delays"=[1000], "PF Delays"=[1000], "Measur. Delays"=[1000.0], "Reject Delays"=[1000], "BF Delays"=[1000]} ("Auto Para"), "Agitator Delays"=w614, "TF Delays"=w612, "Insertion Delays"=w610, "Cutting Delays"=w608, "PF Delays"=w606, "Measur. Delays"=w604, "Reject Delays"=w602, "BF Delays"=w600) -> (w599:T2)
        n254 = Bundle("Auto Para"=w599, "General Para"="General Para") -> (w596:cluster{"Auto Para":T2, "General Para":T1})  [unwired: 1 in]
        n255 = property on="Auto Para" class="Clust (strict)"("Value"=w599) -> ()  [unwired: 2 in, 2 out]
        n256 = call-poly "Enqueue Message.vi"("Message Data"=w596, "Message"="Update Para", "Message Queue"=w594) -> ("error out"=w597:errorcluster, "dup Message Queue"=w593:refnum<queue>)  [unwired: 7 in]
      }
      event "Insertion Para.Delay 1", "Insertion Para.Delay 2", "Agitator Para.Delay 1", "Agitator Para.Delay 2", "Cutting Para.Delay", "Cutting Para.Delay 2", "Cutting Para.Delay 3", "Tube Feeder Para.Delay", "Tube Feeder Para.Delay 2", "Tube Feeder Para.Max Attempts", "PF Para.Delay 1", "PF Para.Delay 2", "Reject Para.Delay", "BF Para.Delay 1", "BF Para.Delay 2", "Tube Feeder Para.Timeout": Mouse Up {
        n257 = event-data() -> ("CtlRef"=w617:refnum<vi>)  [unwired: 1 in, 4 out]
        n258 = property class="DigNum (strict)"(reference=w617) -> (reference out=w620:refnum<vi>, "Value"=w621:u32)  [unwired: 1 in, 1 out]
        n259 = Number To Fractional String(number=w621, precision (6)=0.0 ("width (-)")) -> (F-format string=w619:string)  [unwired: 2 in]
        n260 = call "HMI Pop Up Num KP v1.1.vi"("String In"=w619) -> ("String Out"=w618:string)  [unwired: 9 in, 1 out]
        n261 = Fract/Exp String To Number(string=w618, default (0 dbl)=0.0 ("default (0 I32)")) -> (number=w623:dbl)  [unwired: 2 in, 1 out]
        n262 = property class="DigNum (strict)"(reference=w620, "Value"=w623) -> ()  [unwired: 1 in, 2 out]
      }
      event "Meas. Para.Delay": Mouse Up {
        n263 = event-data() -> ("CtlRef"=w626:refnum<vi>)  [unwired: 1 in, 4 out]
        n264 = property class="DigNum (strict)"(reference=w626) -> (reference out=w629:refnum<vi>, "Value"=w630:dbl)  [unwired: 1 in, 1 out]
        n265 = Number To Fractional String(number=w630, precision (6)=0.0 ("width (-)")) -> (F-format string=w628:string)  [unwired: 2 in]
        n266 = call "HMI Pop Up Num KP v1.1.vi"("String In"=w628) -> ("String Out"=w627:string)  [unwired: 9 in, 1 out]
        n267 = Fract/Exp String To Number(string=w627, default (0 dbl)=0.0 ("default (0 I32)")) -> (number=w632:dbl)  [unwired: 2 in, 1 out]
        n268 = property class="DigNum (strict)"(reference=w629, "Value"=w632) -> ()  [unwired: 1 in, 2 out]
      }
      event "Meas. Para.Mean Length", "Meas. Para.Tolerance": Mouse Up {
        n269 = event-data() -> ("CtlRef"=w635:refnum<vi>)  [unwired: 1 in, 4 out]
        n270 = property class="DigNum (strict)"(reference=w635) -> (reference out=w638:refnum<vi>, "Value"=w639:dbl)  [unwired: 1 in, 1 out]
        n271 = Number To Fractional String(number=w639, precision (6)=2.0 ("width (-)")) -> (F-format string=w637:string)  [unwired: 2 in]
        n272 = call "HMI Pop Up Num KP v1.1.vi"("String In"=w637) -> ("String Out"=w636:string)  [unwired: 9 in, 1 out]
        n273 = Fract/Exp String To Number(string=w636, default (0 dbl)=0.0 ("default (0 I32)")) -> (number=w641:dbl)  [unwired: 2 in, 1 out]
        n274 = property class="DigNum (strict)"(reference=w638, "Value"=w641) -> ()  [unwired: 1 in, 2 out]
      }
      event User Event {
        # "The Message Handling Loop processed an \"Exit\" message, which fired this event to stop the Event Handling Loop."
        n275 = event-data() -> ()  [unwired: 1 in, 1 out]
      }
    }
    n276 = call "Error Handler - Event Handling Loop.vi"("error in (no error)"=w487, "Message Queue"=w485) -> ("dup error in"=w484:errorcluster)  [unwired: 8 in, 1 out]
  }
  n277 = call "HMI-cRIO Connection Manager.vi"("error in"=w2, "notifier in"=w8, "Queue in"=w34) -> ("error out"=w28:errorcluster, "Notifier out"=w29:refnum<notifier>)  [unwired: 7 in]
  n278 = Unregister For Events(event registration refnum=w40, error in=w38) -> (error out=w41:errorcluster)
  n279 = Merge Errors(w41, w43, w28) -> (w42:errorcluster)
  n280 = call "Destroy User Event - Stop.vi"("error in (no error)"=w42, "User Event - Stop"=w36) -> ("error out"=w31:errorcluster)  [unwired: 9 in]
  n281 = Release Notifier(notifier=w29, error in (no error)=w31) -> (error out=w30:errorcluster)  [unwired: 1 in, 2 out]
  n282 = disable-structure shown="RUN_TIME_ENGINE==True" {
    disable-tunnel: w30 -> [_ _]
    frame condition #0 (active) {
    }
    frame condition #1 {
      n283 = local read "Shutdown?"() -> (w646:bool)
      n284 = case shown="True" w646 {
        tunnel: [_ w648] -> w647
        frame False {
        }
        frame True {
          n285 = call <vilib>:"System Exec.vi"("wait until completion? (T)"=TRUE, "command line"="Shutdown -s -f -t 10") -> ("error out"=w648:errorcluster)  [unwired: 6 in, 3 out]
        }
      }
      n286 = flat-sequence {
        tunnel: w647 -> [_]
        frame #0 {
          n287 = Quit LabVIEW() -> ()  [unwired: 1 in]
        }
      }
    }
  }
